vi "IV_measure_DMM.vi"(8 "error in (no error)":errorcluster, 11 "Input parameters":T1={"Measurement type"=enum."Debug", "Sensor type"=enum."HPK_8in_256ch", "Identifier"="test.txt", "Open after execution?"=FALSE, "Plot after execution?"=FALSE, "Display channel"=0, "Voltage Delay (s)"=0.5, "Switch Delay (s)"=0.01, "VISA resource name source"="", "VISA resource name DMM"="", "VISA resource name LCR"="", "Compliance  Level (A)"=10.0, "Voltage Limit (V)"=1000.0, "Data storage location"="", "Scan voltages"="", "Use source as DMM?"=FALSE, "LCR signal frequenzy (Hz)"=10.0, "DMM device"=enum."Keithley2001", "Sampling number"=1, "Use env. sensors on"=enum."Sensirion sht1x/7x", "Switchboard Handle"=0, "Use Switchboard"=FALSE, "LCR signal voltage (V)"=10000.0, "Repeat"=1, "Scan voltages IV"="", "Scan voltages CV"="", "Hex pad numbers?"=FALSE, "Set measurement type"=enum."Debug", "Custom pad scan"="", "IV voltage Delay (s)"=0.5, "CV voltage Delay (s)"=0.5, "Needle measurement?"=FALSE, "Comments"="test.txt", "LCR signal frequenzy (kHz)"=10.0, "Compliance  Level (uA)"=10.0, "Open Correction Array"=array2304x3[6912 elements], "Current set voltage"=0.0, "Last set voltage"=0.0, "Current channel"=0, "Last OpenCorrection index"=-1, "Total curr/vltg every x steps"=10, "Current channel iteration"=0, "No CV corrections"=FALSE, "Mapfile"="", "Corrfile"="", "IV voltage file"=path "", "CV voltage file"=path "", "IV Switch Delay (s)"=0.01, "CV Switch Delay (s)"=0.01, "Invert polarity"=FALSE, "Set debug dirs"=FALSE, "Is n on p"=FALSE, "Source interlock?"=TRUE, "Voltage file used?"=FALSE} {"CV Switch Delay (s)" format="%#_13g"; "IV Switch Delay (s)" format="%#_13g"; "Last set voltage" format="%#_13g"; "Current set voltage" format="%#_13g"; "CV voltage Delay (s)" format="%#_13g"; "IV voltage Delay (s)" format="%#_13g"; "Voltage Limit (V)" format="%#_13g"; "Voltage Delay (s)" format="%#_13g"; "Switch Delay (s)" format="%#_13g"}) -> (0 "error out":errorcluster, 1 "Error":dbl, 2 "Result":dbl, 3 "Input parameters out":T1={"Measurement type"=enum."Debug", "Sensor type"=enum."HPK_8in_256ch", "Identifier"="test.txt", "Open after execution?"=FALSE, "Plot after execution?"=FALSE, "Display channel"=0, "Voltage Delay (s)"=0.5, "Switch Delay (s)"=0.01, "VISA resource name source"="", "VISA resource name DMM"="", "VISA resource name LCR"="", "Compliance  Level (A)"=10.0, "Voltage Limit (V)"=1000.0, "Data storage location"="", "Scan voltages"="", "Use source as DMM?"=FALSE, "LCR signal frequenzy (Hz)"=10.0, "DMM device"=enum."Keithley2001", "Sampling number"=1, "Use env. sensors on"=enum."Sensirion sht1x/7x", "Switchboard Handle"=0, "Use Switchboard"=FALSE, "LCR signal voltage (V)"=10000.0, "Repeat"=1, "Scan voltages IV"="", "Scan voltages CV"="", "Hex pad numbers?"=FALSE, "Set measurement type"=enum."Debug", "Custom pad scan"="", "IV voltage Delay (s)"=0.5, "CV voltage Delay (s)"=0.5, "Needle measurement?"=FALSE, "Comments"="test.txt", "LCR signal frequenzy (kHz)"=10.0, "Compliance  Level (uA)"=10.0, "Open Correction Array"=array2304x3[6912 elements], "Current set voltage"=0.0, "Last set voltage"=0.0, "Current channel"=0, "Last OpenCorrection index"=-1, "Total curr/vltg every x steps"=10, "Current channel iteration"=0, "No CV corrections"=FALSE, "Mapfile"="", "Corrfile"="", "IV voltage file"=path "", "CV voltage file"=path "", "IV Switch Delay (s)"=0.01, "CV Switch Delay (s)"=0.01, "Invert polarity"=FALSE, "Set debug dirs"=FALSE, "Is n on p"=FALSE, "Source interlock?"=TRUE, "Voltage file used?"=FALSE} {"CV Switch Delay (s)" format="%#_13g"; "IV Switch Delay (s)" format="%#_13g"; "Last set voltage" format="%#_13g"; "Current set voltage" format="%#_13g"; "CV voltage Delay (s)" format="%#_13g"; "IV voltage Delay (s)" format="%#_13g"; "Voltage Limit (V)" format="%#_13g"; "Voltage Delay (s)" format="%#_13g"; "Switch Delay (s)" format="%#_13g"})   [LabVIEW 2016]
doc: "Measure current from DMM."
uses:
  input_params.ctl
  <instrlib>/Keithley 2450/Keithley 2450.lvlib
  <instrlib>/Keithley 24XX/Keithley 24XX.lvlib
  <instrlib>/Keithley 6517/Keithley 6517.lvlib
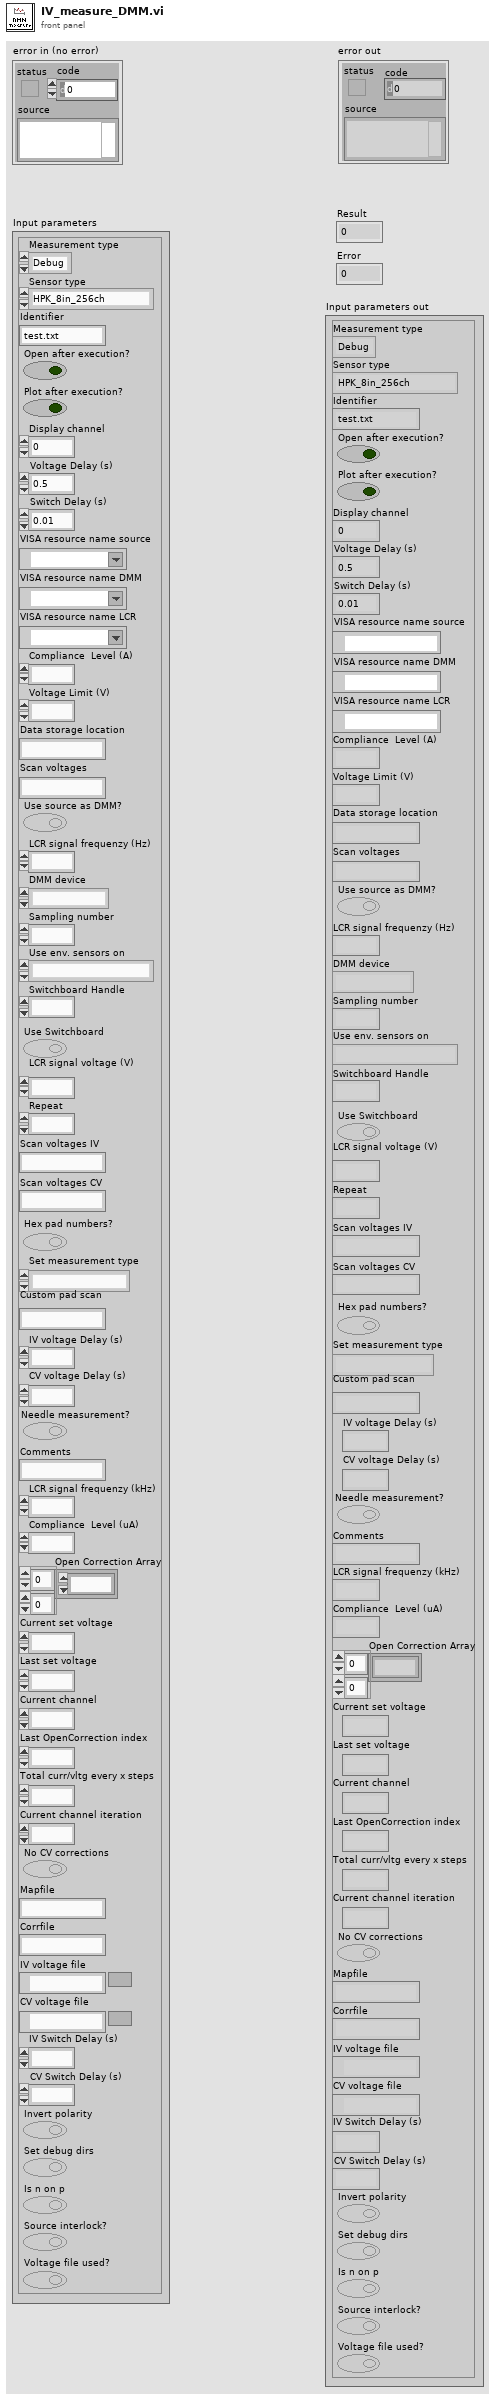
[diagram p1: front panel]
types:
  T1 = typedef "input_params.ctl" = cluster{"Measurement type":enum16{"IV", "CV", "Debug", "Test_contact"}, "Sensor type":enum16{"HPK_6in_135ch", "HPK_8in_256ch", "IFX_8in_256ch", "Diode", "HPK_6in_256ch", "Full_Matrix", ""}, "Identifier":string, "Open after execution?":bool, "Plot after execution?":bool, "Display channel":i32, "Voltage Delay (s)":dbl, "Switch Delay (s)":dbl, "VISA resource name source":refnum<visa-resource-name>, "VISA resource name DMM":refnum<visa-resource-name>, "VISA resource name LCR":refnum<visa-resource-name>, "Compliance  Level (A)":dbl, "Voltage Limit (V)":dbl, "Data storage location":string, "Scan voltages":string, "Use source as DMM?":bool, "LCR signal frequenzy (Hz)":dbl, "DMM device":enum16{"Keithley2001", "Keithley2450", "Keithley2410", "Keithley6487", "Keithley6517"}, "Sampling number":i32, "Use env. sensors on":enum16{"Sensirion sht1x/7x", "Switch Matrix", "Probecard"}, "Switchboard Handle":u32, "Use Switchboard":bool, "LCR signal voltage (V)":dbl, "Repeat":i32, "Scan voltages IV":string, "Scan voltages CV":string, "Hex pad numbers?":bool, "Set measurement type":enum16{"IV", "CV", "Debug", "Test_contact", "IV+CV"}, "Custom pad scan":string, "IV voltage Delay (s)":dbl, "CV voltage Delay (s)":dbl, "Needle measurement?":bool, "Comments":string, "LCR signal frequenzy (kHz)":dbl, "Compliance  Level (uA)":dbl, "Open Correction Array":dbl[][], "Current set voltage":dbl, "Last set voltage":dbl, "Current channel":i32, "Last OpenCorrection index":i32, "Total curr/vltg every x steps":i32, "Current channel iteration":i32, "No CV corrections":bool, "Mapfile":string, "Corrfile":string, "IV voltage file":path, "CV voltage file":path, "IV Switch Delay (s)":dbl, "CV Switch Delay (s)":dbl, "Invert polarity":bool, "Set debug dirs":bool, "Is n on p":bool, "Source interlock?":bool, "Voltage file used?":bool}
  T2 = enum16{"Keithley2001", "Keithley2450", "Keithley2410", "Keithley6487", "Keithley6517"}
  T3 = cluster{"error":bool, "code":i32, "source":string}
  T4 = cluster{"Measurement":dbl, "Units":string, "Time Stamp and Date":string, "Reading #":dbl, "Channel #":dbl}
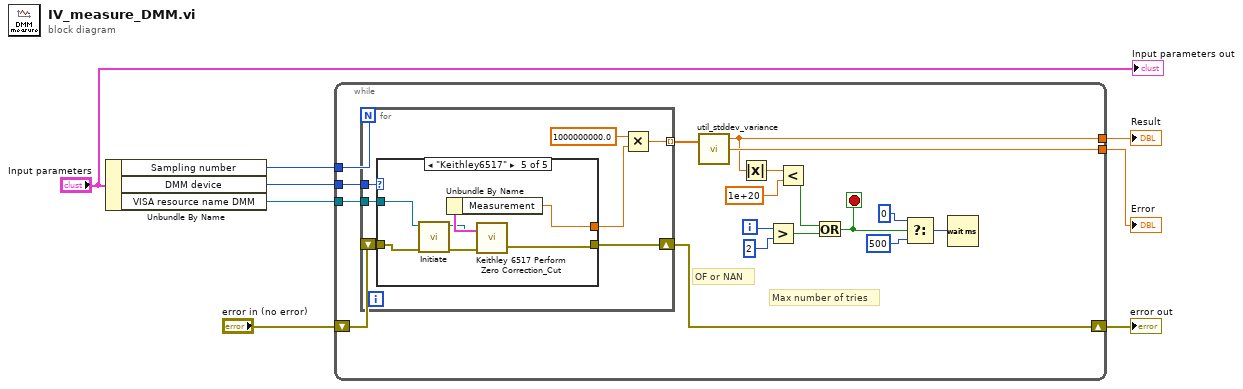
[diagram p0: block diagram]
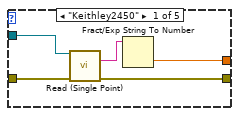
[diagram p2: hidden frame]
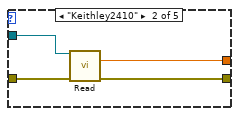
[diagram p3: hidden frame]
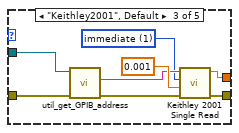
[diagram p4: hidden frame]
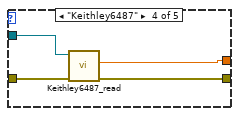
[diagram p5: hidden frame]
diagram:
  n1 = Unbundle By Name("Input parameters") -> ("Sampling number"=w4:i32, "DMM device"=w7:T2, "VISA resource name DMM"=w6:refnum<visa-resource-name>)
  n2 = while {
    tunnel: w7 -> [w25]
    tunnel: w6 -> [w24]
    tunnel: w4 -> [w22]
    tunnel: [w20] -> w3
    tunnel: [w19] -> w1
    shift-right: [w26] -> w8
    shift-left: "error in (no error)" -> [w23]
    i -> [w14]
    stop <- w12 stop-if-true
    # "OF or NAN"
    # "Max number of tries"
    n3 = for {
      N: w22 -> [_]
      tunnel: w25 -> [w32]
      tunnel: w24 -> [w31]
      tunnel: [w27] -> w21 mode=indexing
      shift-right: [w33] -> w26
      shift-left: w23 -> [w30]
      n4 = case shown="\"Keithley6517\"" w32 {
        tunnel: w30 -> [w37 w42 w47 w52 w58]
        tunnel: w31 -> [w36 w39 w44 w53 w57]
        tunnel: [w35 w41 w50 w51 w55] -> w33
        tunnel: [w34 w40 w48 w54 w56] -> w28
        frame "Keithley2450" {
          n5 = call <instrlib>:"Read (Single Point).vi"("VISA resource name"=w36, "error in (no error)"=w37) -> ("Data out"=w38:string, "error out"=w35:errorcluster)  [unwired: 11 in, 1 out]
          n6 = Fract/Exp String To Number(string=w38) -> (number=w34:dbl)  [unwired: 3 in, 1 out]
        }
        frame "Keithley2410" {
          n7 = call-poly <instrlib>:"Read.vi"("VISA resource name"=w39, "error in (no error)"=w42) -> ("Current"=w40:sgl, "error out"=w41:errorcluster)  [unwired: 7 in, 5 out]
        }
        frame "Keithley2001", Default {
          w43 = u16 1 items=["hold", "immediate", "timer", "manual", "bus", "trigger link", "external"] ("source (imm:1)")
          n8 = call "util_get_GPIB_address.vi"("error in (no error)"=w47, "VISA resource name"=w44) -> ("error out"=w46:errorcluster, "GPIB address"=w45:string)  [unwired: 7 in, 1 out]
          n9 = call <instrlib>:"Keithley 2001 Single Read.vi"("GPIB address"=w45, "source (imm:1)"=w43, "timer value (secs)"=0.001, "error in"=w46) -> ("measurement"=w48:dbl, "error out"=w50:T3)  [unwired: 4 out]
        }
        frame "Keithley6487" {
          n10 = call <instrlib>:"Keithley6487_read.vi"("error in (no error)"=w52, "VISA resource name"=w53) -> ("error out"=w51:errorcluster, "output"=w54:dbl)  [unwired: 7 in, 1 out]
        }
        frame "Keithley6517" {
          n11 = call <instrlib>:"Initiate.vi"("error in (no error)"=w58, "VISA resource name"=w57) -> ("error out"=w60:errorcluster, "VISA resource name out"=w59:refnum<visa-resource-name>)  [unwired: 8 in]
          n12 = call <instrlib>:"Keithley 6517 Perform Zero Correction_Cut.vi"("Error In"=w60, "VISA resource name"=w59) -> ("Error Out"=w55:errorcluster, "Measurement"=w61:T4)
          n13 = Unbundle By Name(w61) -> ("Measurement"=w56:dbl)
        }
      }
      n14 = Multiply(x=1000000000.0, y=w28) -> (x*y=w27:dbl)
    }
    n15 = call "util_stddev_variance.vi"("X"=w21) -> ("mean"=w19:dbl, "standard deviation"=w20:dbl)  [unwired: 1 in, 1 out]
    n16 = Absolute Value(x=w19) -> (abs(x)=w18:dbl)
    n17 = Greater?(x=w14, y=2) -> (0:w16:bool)
    n18 = Less?(x=w18, y=1e+20) -> (x < y?=w15:bool)
    n19 = Or(x=w15, y=w16) -> (x .or. y?=w12:bool)
    n20 = Select(t=0, s=w12, f=500) -> (s? t:f=w10:i32)
    n21 = Wait (ms)(milliseconds to wait=w10) -> ()  [unwired: 1 out]
  }
  "error out" <- w8
  "Result" <- w1
  "Error" <- w3
  "Input parameters out" <- "Input parameters"
